vi "Init Hardware.vi"(8 "error in (no error)":errorcluster, 11 "Arduino Temperature Controller Driver in":refnum<class "Arduino Temperature Controller Driver.lvclass">) -> (0 "error out":errorcluster, 3 "Arduino Temperature Controller Driver out":refnum<class "Arduino Temperature Controller Driver.lvclass">)   [LabVIEW 2019, in "Arduino Temperature Controller Driver.lvclass"]
uses:
  Arduino Temperature Controller Driver.lvclass
  C:/GitHub/NHMFL_Core/Libraries/Instruments/VISA Instrument/VISA Instrument.lvclass
  VISA Instrument/VISA Instrument.lvclass/VISA Instrument.ctl
  VISA Instrument/Read VISA resource.vi
  VISA Instrument/Write VISA resource.vi
  Temperature Controller Driver/Temperature Controller Driver.lvclass
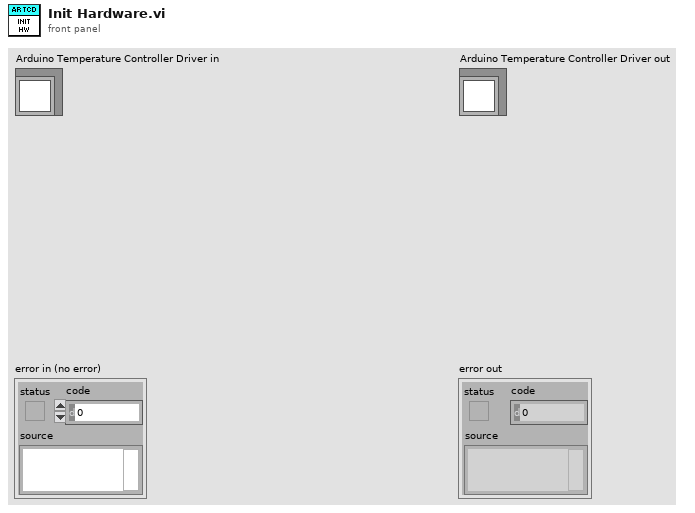
[diagram p1: front panel]
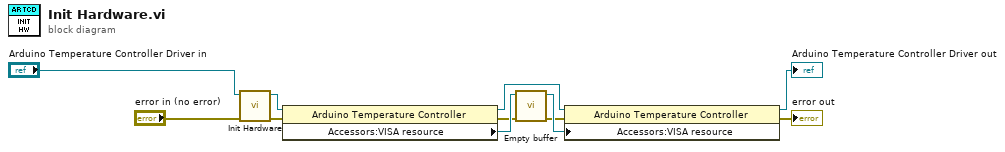
[diagram p0: block diagram]
diagram:
  n1 = call-parent "Init Hardware.vi"("error in (no error)"="error in (no error)", "Temperature Controller Driver in"="Arduino Temperature Controller Driver in") -> ("error out"=w11:errorcluster, "Temperature Controller Driver out"=w8:refnum<class "Arduino Temperature Controller Driver.lvclass">)  [unwired: 8 in]
  n2 = property class="Arduino Temperature Controller "(reference=w8, error in=w11) -> (reference out=w5:refnum<class "Arduino Temperature Controller Driver.lvclass">, error out=w2:errorcluster, "Accessors:VISA resource"=w7:refnum<visa-resource-name>)
  n3 = call "Empty buffer.vi"("Error In"=w2, "VISA resource name"=w7) -> ("Error Out"=w1:errorcluster, "VISA resource name out"=w3:refnum<visa-resource-name>)  [unwired: 7 in, 1 out]
  n4 = property class="Arduino Temperature Controller "(reference=w5, error in=w1, "Accessors:VISA resource"=w3) -> (reference out=→"Arduino Temperature Controller Driver out":refnum<class "Arduino Temperature Controller Driver.lvclass">, error out=→"error out":errorcluster)
